vi "Close.vi"(8 "Error":errorcluster, 11 "Tree in":refnum<class "Tree.lvclass">) -> (0 "Error":errorcluster, 2 "TopVisible":string, 3 "TreeItems[]":T1(array[cluster]))   [LabVIEW 2021, in "Tree.lvlib" / "Tree.lvclass"]
uses:
  Tree.lvclass
  Private/TreeControllerTag.ctl
  Tree.lvclass/Tree.ctl
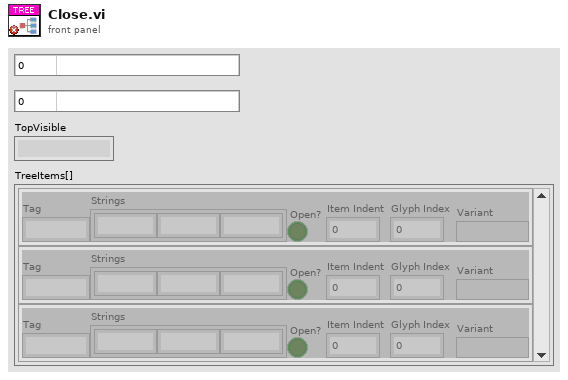
[diagram p1: front panel]
types:
  T1 = cluster{"Tag":string, "Strings":string[], "Open?":bool, "Item Indent":i32, "Glyph Index":i32, "Variant":variant}[]
  T2 = typedef "Tree.lvlib/Tree.lvclass/TreeControllerTag.ctl" = enum8{"Null", "1. Add item", "2. Delete item", "3. Get All Tree Data", "4. Drag Starting", "5. Drag Ended", "6. Add Tree Values", "7. Get Item Value", "8. Edit Item", "9. StepBack", "10. Filter"}
  T3 = cluster{"Node":string, cluster{"Tag":string, "Strings":string[], "Open?":bool, "Item Indent":i32, "Glyph Index":i32, "Variant":variant}[]}
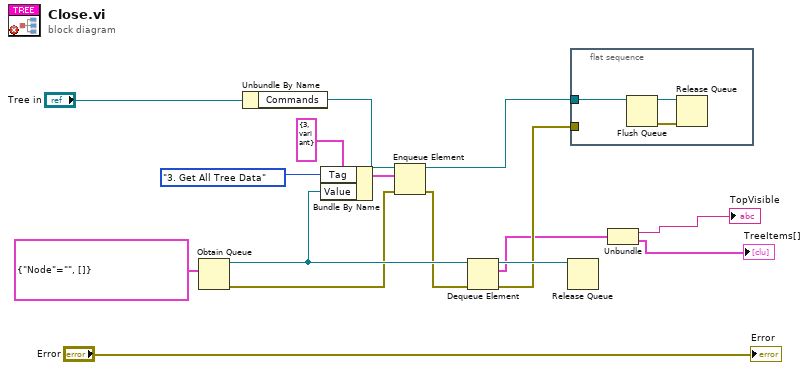
[diagram p0: block diagram]
diagram:
  n1 = Obtain Queue(element data type=T3 {"Node"="", []} ("output cluster")) -> (queue out=w11:refnum<queue>, error out=w7:errorcluster)  [unwired: 4 in, 1 out]
  n2 = Unbundle By Name("Tree in") -> ("Commands"=w14:refnum<queue>)
  n3 = Bundle By Name(cluster=cluster{"Tag":u8, "Value":variant} {"Tag"=3, "Value"=variant} ("element"), "Tag"=TreeControllerTag."3. Get All Tree Data", "Value"=w11) -> (w12:cluster{"Tag":u8, "Value":variant})
  n4 = Enqueue Element(queue=w14, element=w12, error in (no error)=w7) -> (queue out=w9:refnum<queue>, error out=w8:errorcluster)  [unwired: 1 in, 1 out]
  n5 = Dequeue Element(queue=w11, error in (no error)=w8) -> (queue out=w10:refnum<queue>, element=w4:T3, error out=w6:errorcluster)  [unwired: 1 in, 1 out]
  n6 = Release Queue(queue=w10) -> ()  [unwired: 2 in, 3 out]
  n7 = flat-sequence {
    tunnel: w9 -> [w18]
    tunnel: w6 -> [_]
    frame #0 {
      n8 = Flush Queue(queue=w18) -> (queue out=w19:refnum<queue>, error out=w17:errorcluster)  [unwired: 1 in, 1 out]
      n9 = Release Queue(queue=w19, error in (no error)=w17) -> ()  [unwired: 1 in, 3 out]
    }
  }
  n10 = Unbundle(w4) -> ("Node"=→"TopVisible":string, →"TreeItems[]":T1)
  "Error" <- "Error"
